vi "Unflatten.vi"(8 "error in (no error)":errorcluster, 9 "Timeout":bool, 10 "DAQ In":T1[](array[typedef]), 11 "CIF_NIChn_FIFO_DAQ in":refnum<class "CIF_NIChn_Fifo_DAQ.lvclass">) -> (0 "error out":errorcluster, 1 "Header":T2, 2 "DAQ Out":T1[](array[typedef]), 3 "CIF_NIChn_FIFO_DAQ out":refnum<class "CIF_NIChn_Fifo_DAQ.lvclass">)   [LabVIEW 2021, in "CIF_NIChn_FIFO_DAQ.lvclass"]
uses:
  FIFO_DAQ - Copy/CIF_NIChn_Fifo_DAQ.lvclass
  4ab41953-a001-49d2-beab-55370b6c3c42.vi
  7cd889b7-face-4678-a9e3-2692853b6930.vi
  CIFChannels/CIFChannels.lvclass
  CIF_NIChn_FIFO_DAQ.lvclass
  D:/dev/Packages/Channel_Manager/src/CIF_NIChn/NIChn/CIF_NIChn.lvclass
  D:/dev/Packages/Channel_Manager/src/CIFChannels/CIFChannels.lvclass
  D:/dev/Packages/Channel_Manager/src/CIF_NIChn/Archive/FIFO_DAQ - Copy/CIF_NIChn_Fifo_DAQ.lvclass
  ChannelCommon/typedef/FIFO Header.ctl
  ChannelCommon/ChannelCommon.lvlib
  ChannelCommon/typedef/Datatype Waveform.ctl
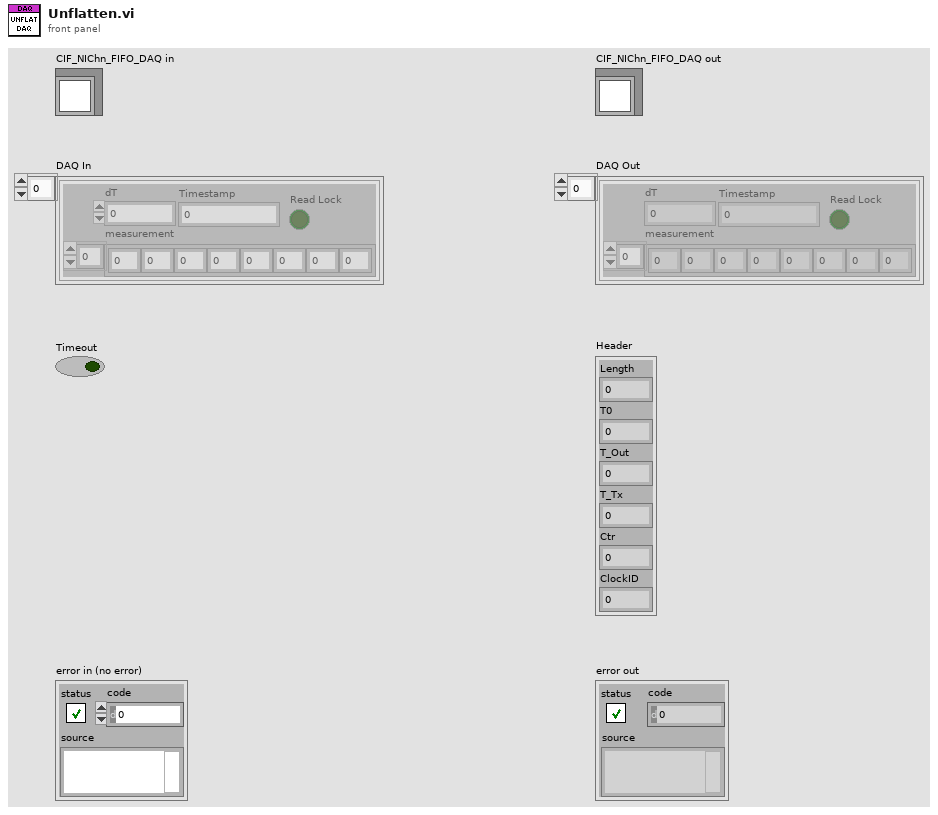
[diagram p1: front panel]
types:
  T1 = typedef "ChannelCommon.lvlib/Datatype Waveform.ctl" = cluster{"measurement":dbl[], "dT":dbl, "Timestamp":i64, "Read Lock":bool}
  T2 = typedef "ChannelCommon.lvlib/FIFO Header.ctl" = cluster{"Length":u64, "T0":i64, "T_Out":i64, "T_Tx":i64, "Ctr":u64, "ClockID":u8}
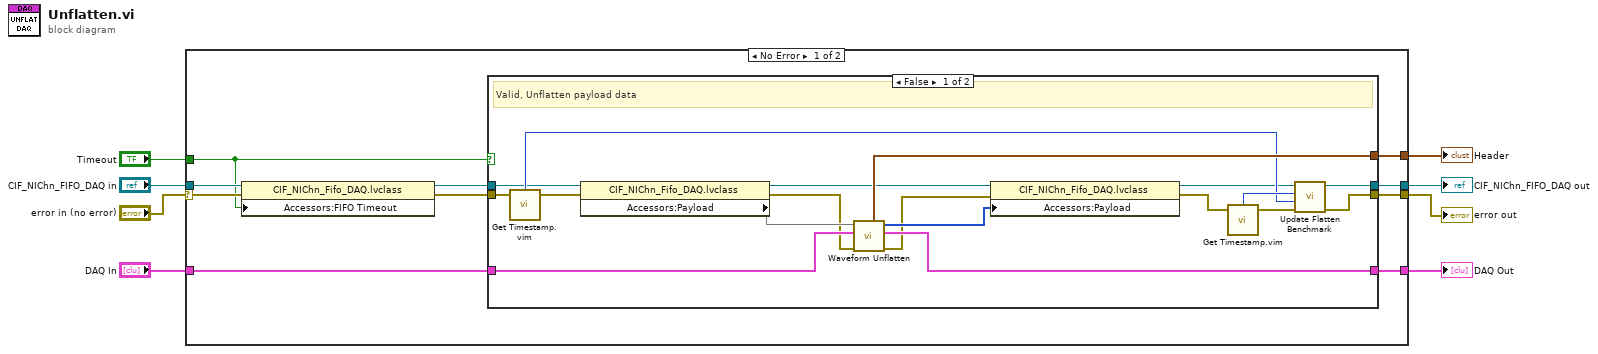
[diagram p0: block diagram]
diagram:
  n1 = case shown="No Error" "error in (no error)" {
    selector: "error in (no error)" -> [w13 w42]
    tunnel: [w16 w42] -> w5
    tunnel: [w17 w41] -> w6
    tunnel: "CIF_NIChn_FIFO_DAQ in" -> [w12 w41]
    tunnel: [w18 _] -> w7
    tunnel: "Timeout" -> [w11 _]
    tunnel: "DAQ In" -> [w10 w40]
    tunnel: [w9 w40] -> w8
    frame No Error {
      n2 = property class="CIF_NIChn_Fifo_DAQ.lvclass"(reference=w12, error in=w13, "Accessors:FIFO Timeout"=w11) -> (reference out=w15:refnum<class "CIF_NIChn_Fifo_DAQ.lvclass">, error out=w14:errorcluster)
      n3 = case shown="False" w11 {
        tunnel: w14 -> [w36 w38]
        tunnel: w15 -> [w27 w39]
        tunnel: [w31 _] -> w18
        tunnel: [w35 w39] -> w17
        tunnel: [w34 w38] -> w16
        tunnel: w10 -> [w33 w37]
        tunnel: [w32 w37] -> w9
        frame False {
          # "Valid, Unflatten payload data"
          n4 = call "Get Timestamp.vim"("Anything in"=w36) -> ("Time (ns)"=w29:i64, "Anything out"=w22:errorcluster)  [unwired: 2 in]
          n5 = property class="CIF_NIChn_Fifo_DAQ.lvclass"(reference=w27, error in=w22) -> (reference out=w25:refnum<class "CIF_NIChn_Fifo_DAQ.lvclass">, error out=w21:errorcluster, "Accessors:Payload"=w26)
          n6 = call "Waveform Unflatten.vi"("error in (no error)"=w21, "Data in in"=w33, "Flatten Data in"=w26) -> ("error out"=w20:errorcluster, "Data out"=w32:T1[], "Flatten Data out"=w24:u8[], "Header out"=w31:T2)  [unwired: 5 in]
          n7 = property class="CIF_NIChn_Fifo_DAQ.lvclass"(reference=w25, error in=w20, "Accessors:Payload"=w24) -> (reference out=w23:refnum<class "CIF_NIChn_Fifo_DAQ.lvclass">, error out=w19:errorcluster)
          n8 = call "Get Timestamp.vim"("Anything in"=w19) -> ("Time (ns)"=w30:i64, "Anything out"=w28:errorcluster)  [unwired: 2 in]
          n9 = call "Update Flatten Benchmark.vi"("error in (no error)"=w28, "X0"=w29, "X1"=w30, "CIFChannels in"=w23) -> ("error out"=w34:errorcluster, "CIFChannels out"=w35:refnum<class "CIF_NIChn_Fifo_DAQ.lvclass">)  [unwired: 6 in]
        }
        frame True {
          # "Timeout"
        }
      }
    }
    frame Error {
    }
  }
  "error out" <- w5
  "CIF_NIChn_FIFO_DAQ out" <- w6
  "Header" <- w7
  "DAQ Out" <- w8
